vi "WCA_GET_PA.vi"(0 "Cartridge Band":u32=10, 1 "Slave Node in":cluster{"Address":i16, "Serial Number":i8[]}={"Address"=19, "Serial Number"=[16, 71, 55, 76, 1, 8, 0, -15]} {"Serial Number" format="%.0x"; "Address" format="%.0x"}, 2 "ObjHandle in":u32, 11 "error in (no error)":errorcluster) -> (4 "ObjHandle out":u32=92930112, 8 "GET_PA":T1={"PA_A_DRAIN_V"=0.0051879883, "PA_A_DRAIN_C"=3.829956, "PA_A_GATE_V"=-0.00061035156, "PA_B_DRAIN_V"=0.003967285, "PA_B_DRAIN_C"=4.4555664, "PA_B_GATE_V"=0.0018310547, "PA_3V_SUPPLY_V"=3.7371826, "PA_5V_MON"=5.310364}, 15 "error out":errorcluster)   [LabVIEW 2017]
uses:
  WCA_Global.vi
panel:
  # "Vd [V]"
  # "Id [mA]"
  # "Vg [V]"
  # "PA -3V Supply"
  # "-3V"
  # "PA A"
  # "+5V"
  # "PA B"
  # "Node Address"
  # "Serial Number"
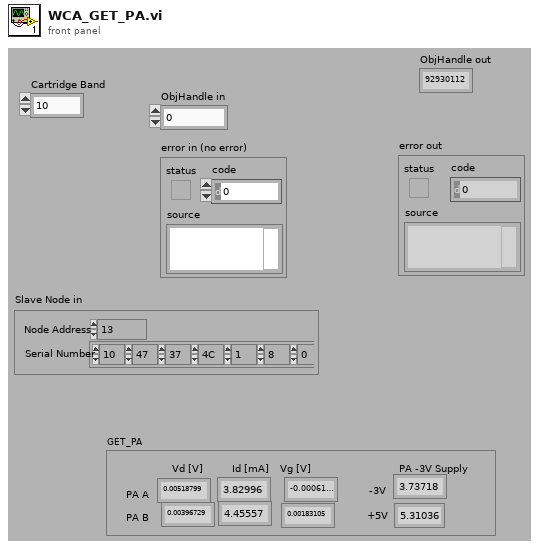
[diagram p1: front panel]
types:
  T1 = cluster{"PA_A_DRAIN_V":sgl, "PA_A_DRAIN_C":sgl, "PA_A_GATE_V":sgl, "PA_B_DRAIN_V":sgl, "PA_B_DRAIN_C":sgl, "PA_B_GATE_V":sgl, "PA_3V_SUPPLY_V":sgl, "PA_5V_MON":sgl}
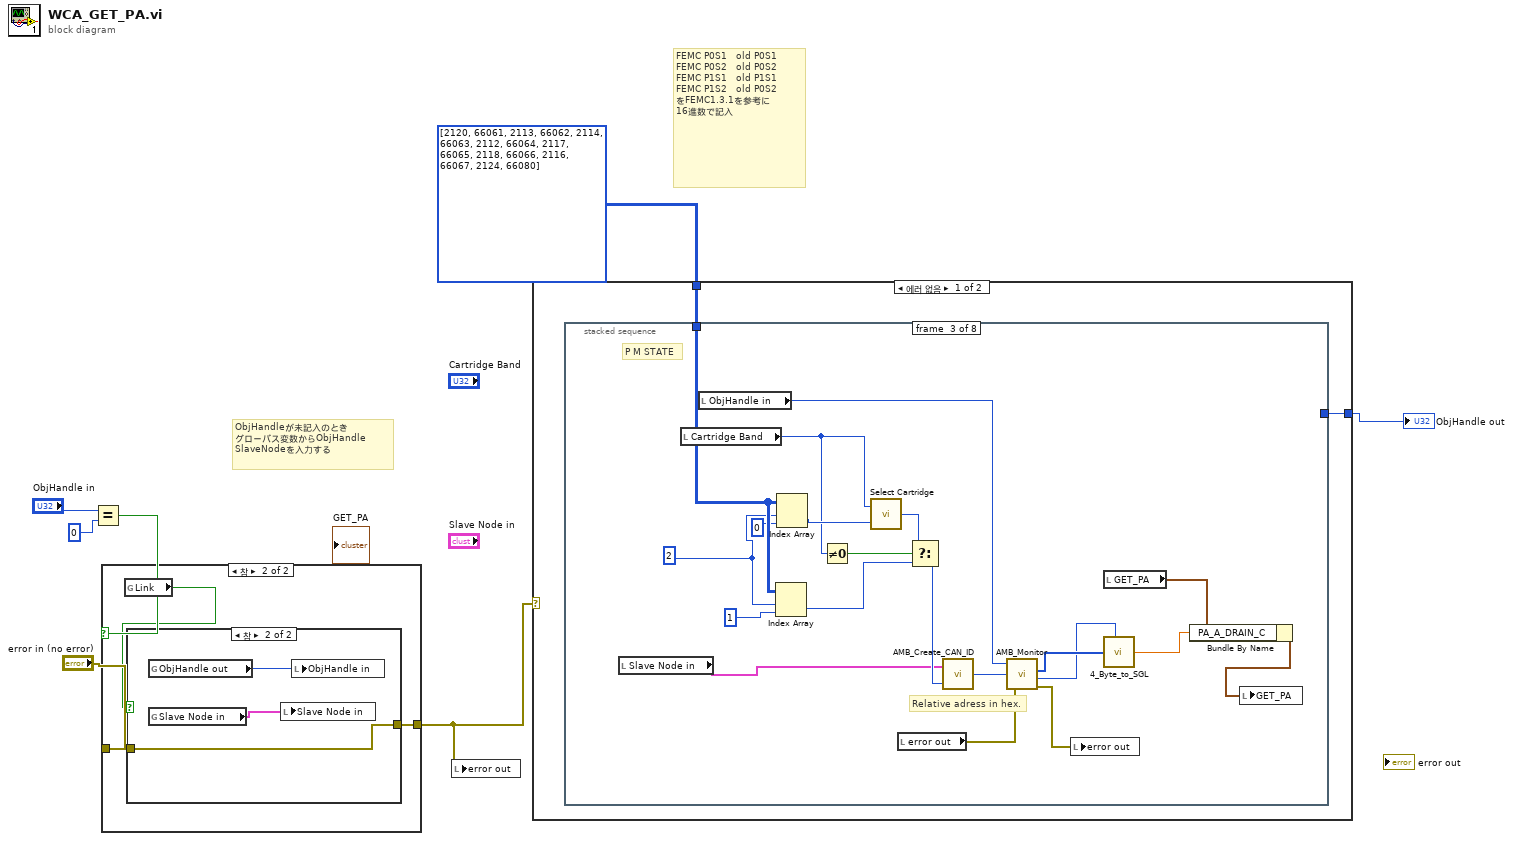
[diagram p0: block diagram]
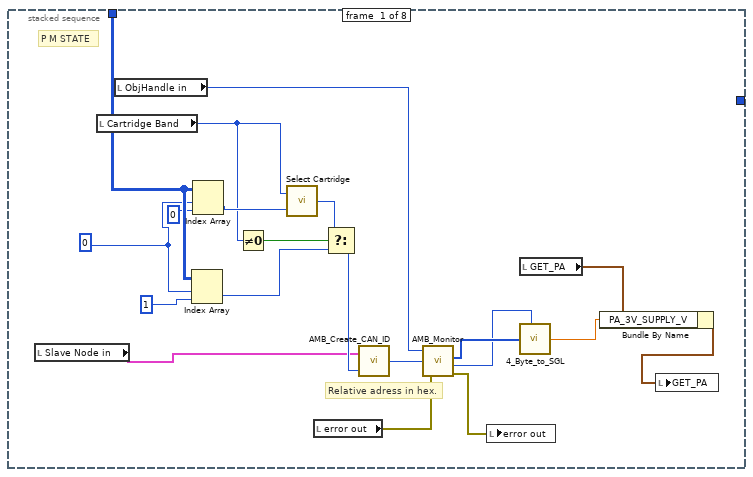
[diagram p2: hidden frame]
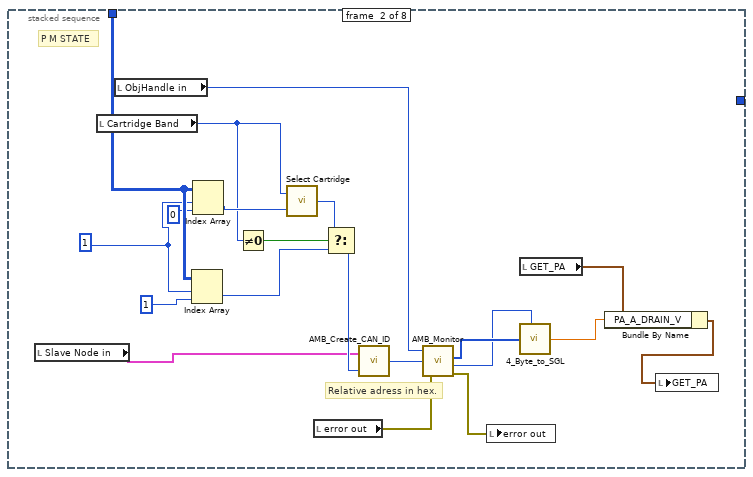
[diagram p3: hidden frame]
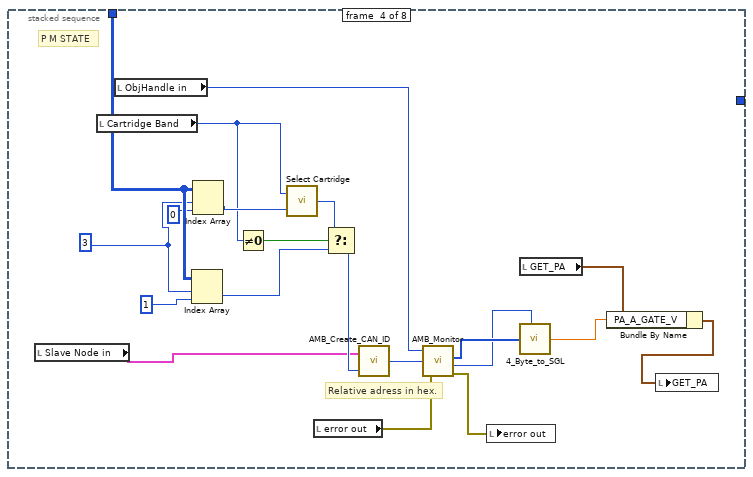
[diagram p4: hidden frame]
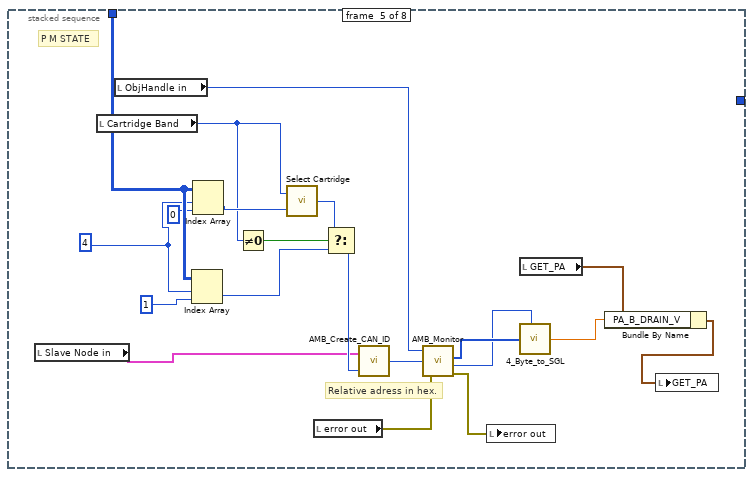
[diagram p5: hidden frame]
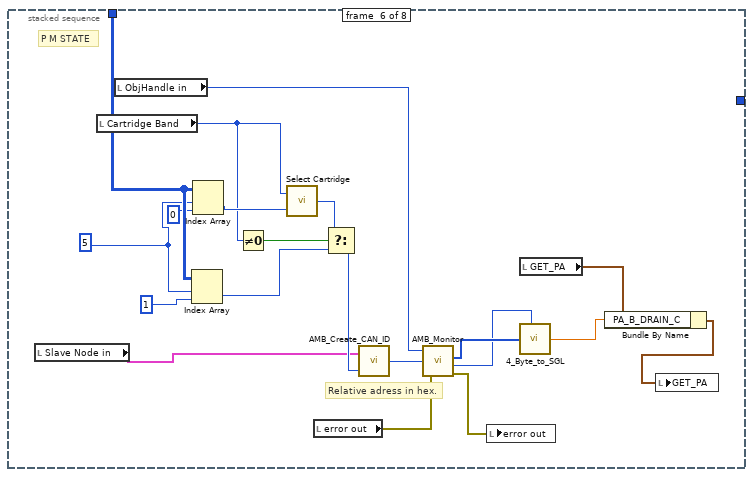
[diagram p6: hidden frame]
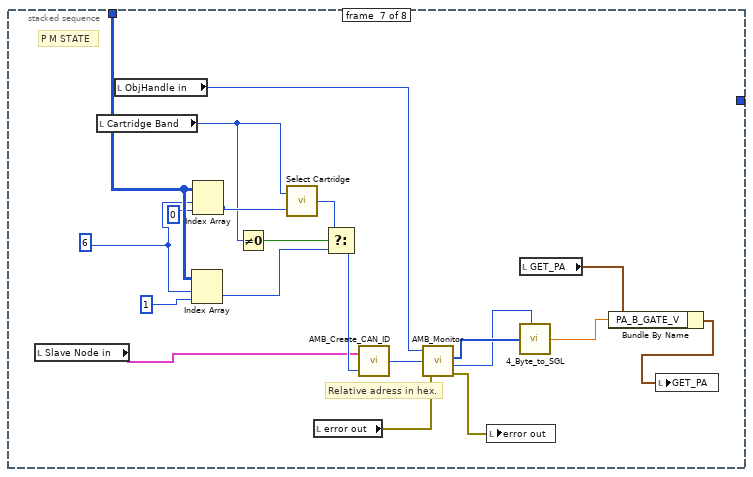
[diagram p7: hidden frame]
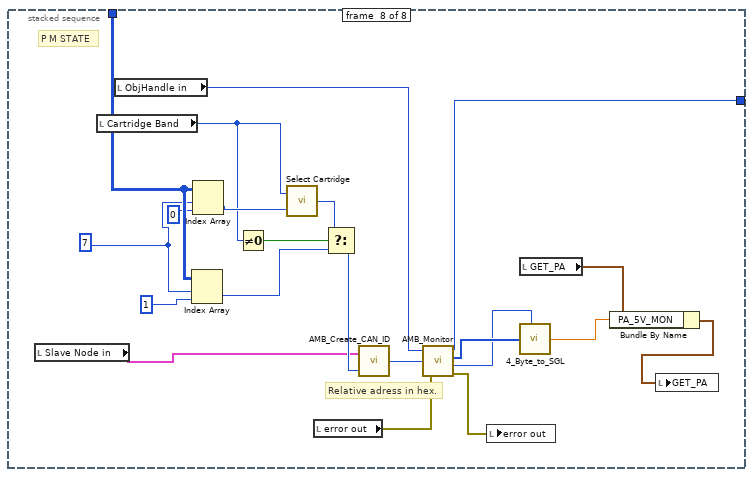
[diagram p8: hidden frame]
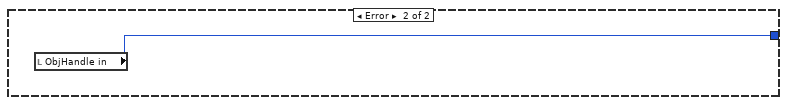
[diagram p9: hidden frame]
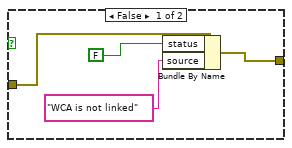
[diagram p11: hidden frame]
diagram:
  # "ObjHandleが未記入のとき\nグローバス変数からObjHandle\nSlaveNodeを入力する"
  # "FEMC P0S1   old P0S1\nFEMC P0S2   old P0S2\nFEMC P1S1   old P1S1\nFEMC P1S2   old P0S2\nをFEMC1.3.1を参考に\n16進数で記入"
  n1 = Equal?(x="ObjHandle in", y=0) -> (x = y?=w5:bool)
  n2 = case shown="참" w5 {
    tunnel: "error in (no error)" -> [w8 w11]
    tunnel: [w8 w10] -> w3
    frame False {
    }
    frame True {
      n3 = global read "WCA_Global.vi" "Link"() -> (w9:bool)
      n4 = case shown="참" w9 {
        tunnel: w11 -> [w15 w16]
        tunnel: [w12 w16] -> w10
        frame False {
          n5 = Bundle By Name(cluster=w15, "status"=FALSE, "source"="WCA is not linked") -> (w12:errorcluster)
        }
        frame True {
          n6 = global read "WCA_Global.vi" "ObjHandle out"() -> (w18:u32)
          n7 = global read "WCA_Global.vi" "Slave Node in"() -> (w17:cluster{"Address":i16, "Serial Number":i8[]})
          n8 = local write "Slave Node in"(w17) -> ()
          n9 = local write "ObjHandle in"(w18) -> ()
        }
      }
    }
  }
  n10 = local write "error out"(w3) -> ()
  n11 = case shown="에러 없음" w3 {
    tunnel: [w19 w182] -> w2
    tunnel: i32[][] [[2120, 66061], [2113, 66062], [2114, 66063], [2112, 66064], [2117, 66065], [2118, 66066], [2116, 66067], [2124, 66080]] -> [w20 _]
    frame No Error {
      n12 = stacked-sequence {
        tunnel: w20 -> [w40 w60 w80 w100 w120 w140 w160 w181]
        tunnel: [_ _ _ _ _ _ _ w161] -> w19
        frame #0 {
          w25 = 0
          # "Relative adress in hex."
          # "P M STATE"
          n13 = local read "Slave Node in"() -> (w24:cluster{"Address":i16, "Serial Number":i8[]})
          n14 = local read "Cartridge Band"() -> (w26:u32)
          n15 = local read "ObjHandle in"() -> (w36:u32)
          n16 = Index Array(array=w40, index (row)=w25, index (col)=1) -> (element=w35:i32)
          n17 = Index Array(array=w40, index (row)=w25, index (col)=0) -> (element=w34:i32)
          n18 = Not Equal To 0?(x=w26) -> (x != 0?=w37:bool)
          n19 = call "Select Cartridge.vi"("Relative Address in"=w34, "Cartridge band"=w26) -> ("Relative Address out"=w38:u32)
          n20 = local read "error out"() -> (w28:errorcluster)
          n21 = Select(t=w38, s=w37, f=w35) -> (s? t:f=w39:u32)
          n22 = call "AMB_Create_CAN_ID.vi"("Relative Address in"=w39, "Slave Node in"=w24) -> ("CAN ID out"=w31:u32)
          n23 = call "AMB_Monitor.vi"("ObjHandle in"=w36, "CAN ID in"=w31, "error in"=w28) -> ("Data Array out"=w23:u8[], "Data Length out"=w22:u8, "error out"=w27:errorcluster)  [unwired: 1 out]
          n24 = local write "error out"(w27) -> ()
          n25 = local read "GET_PA"() -> (w30:T1)
          n26 = call "4_Byte_to_SGL.vi"("Array of 4 bytes"=w23, "number of valid bytes"=w22) -> ("Number"=w21:sgl)  [unwired: 1 out]
          n27 = Bundle By Name(cluster=w30, "PA_3V_SUPPLY_V"=w21) -> (w29:T1)
          n28 = local write "GET_PA"(w29) -> ()
        }
        frame #1 {
          w45 = 1
          # "Relative adress in hex."
          # "P M STATE"
          n29 = local read "Slave Node in"() -> (w44:cluster{"Address":i16, "Serial Number":i8[]})
          n30 = local read "Cartridge Band"() -> (w46:u32)
          n31 = local read "ObjHandle in"() -> (w56:u32)
          n32 = Index Array(array=w60, index (row)=w45, index (col)=1) -> (element=w55:i32)
          n33 = Index Array(array=w60, index (row)=w45, index (col)=0) -> (element=w54:i32)
          n34 = Not Equal To 0?(x=w46) -> (x != 0?=w57:bool)
          n35 = call "Select Cartridge.vi"("Relative Address in"=w54, "Cartridge band"=w46) -> ("Relative Address out"=w58:u32)
          n36 = local read "error out"() -> (w48:errorcluster)
          n37 = Select(t=w58, s=w57, f=w55) -> (s? t:f=w59:u32)
          n38 = call "AMB_Create_CAN_ID.vi"("Relative Address in"=w59, "Slave Node in"=w44) -> ("CAN ID out"=w51:u32)
          n39 = call "AMB_Monitor.vi"("ObjHandle in"=w56, "CAN ID in"=w51, "error in"=w48) -> ("Data Array out"=w43:u8[], "Data Length out"=w42:u8, "error out"=w47:errorcluster)  [unwired: 1 out]
          n40 = local write "error out"(w47) -> ()
          n41 = local read "GET_PA"() -> (w50:T1)
          n42 = call "4_Byte_to_SGL.vi"("Array of 4 bytes"=w43, "number of valid bytes"=w42) -> ("Number"=w41:sgl)  [unwired: 1 out]
          n43 = Bundle By Name(cluster=w50, "PA_A_DRAIN_V"=w41) -> (w49:T1)
          n44 = local write "GET_PA"(w49) -> ()
        }
        frame #2 {
          w65 = 2
          # "Relative adress in hex."
          # "P M STATE"
          n45 = local read "Slave Node in"() -> (w64:cluster{"Address":i16, "Serial Number":i8[]})
          n46 = local read "Cartridge Band"() -> (w66:u32)
          n47 = local read "ObjHandle in"() -> (w76:u32)
          n48 = Index Array(array=w80, index (row)=w65, index (col)=1) -> (element=w75:i32)
          n49 = Index Array(array=w80, index (row)=w65, index (col)=0) -> (element=w74:i32)
          n50 = Not Equal To 0?(x=w66) -> (x != 0?=w77:bool)
          n51 = call "Select Cartridge.vi"("Relative Address in"=w74, "Cartridge band"=w66) -> ("Relative Address out"=w78:u32)
          n52 = local read "error out"() -> (w68:errorcluster)
          n53 = Select(t=w78, s=w77, f=w75) -> (s? t:f=w79:u32)
          n54 = call "AMB_Create_CAN_ID.vi"("Relative Address in"=w79, "Slave Node in"=w64) -> ("CAN ID out"=w71:u32)
          n55 = call "AMB_Monitor.vi"("ObjHandle in"=w76, "CAN ID in"=w71, "error in"=w68) -> ("Data Array out"=w63:u8[], "Data Length out"=w62:u8, "error out"=w67:errorcluster)  [unwired: 1 out]
          n56 = local write "error out"(w67) -> ()
          n57 = local read "GET_PA"() -> (w70:T1)
          n58 = call "4_Byte_to_SGL.vi"("Array of 4 bytes"=w63, "number of valid bytes"=w62) -> ("Number"=w61:sgl)  [unwired: 1 out]
          n59 = Bundle By Name(cluster=w70, "PA_A_DRAIN_C"=w61) -> (w69:T1)
          n60 = local write "GET_PA"(w69) -> ()
        }
        frame #3 {
          w85 = 3
          # "Relative adress in hex."
          # "P M STATE"
          n61 = local read "Slave Node in"() -> (w84:cluster{"Address":i16, "Serial Number":i8[]})
          n62 = local read "Cartridge Band"() -> (w86:u32)
          n63 = local read "ObjHandle in"() -> (w96:u32)
          n64 = Index Array(array=w100, index (row)=w85, index (col)=1) -> (element=w95:i32)
          n65 = Index Array(array=w100, index (row)=w85, index (col)=0) -> (element=w94:i32)
          n66 = Not Equal To 0?(x=w86) -> (x != 0?=w97:bool)
          n67 = call "Select Cartridge.vi"("Relative Address in"=w94, "Cartridge band"=w86) -> ("Relative Address out"=w98:u32)
          n68 = local read "error out"() -> (w88:errorcluster)
          n69 = Select(t=w98, s=w97, f=w95) -> (s? t:f=w99:u32)
          n70 = call "AMB_Create_CAN_ID.vi"("Relative Address in"=w99, "Slave Node in"=w84) -> ("CAN ID out"=w91:u32)
          n71 = call "AMB_Monitor.vi"("ObjHandle in"=w96, "CAN ID in"=w91, "error in"=w88) -> ("Data Array out"=w83:u8[], "Data Length out"=w82:u8, "error out"=w87:errorcluster)  [unwired: 1 out]
          n72 = local write "error out"(w87) -> ()
          n73 = local read "GET_PA"() -> (w90:T1)
          n74 = call "4_Byte_to_SGL.vi"("Array of 4 bytes"=w83, "number of valid bytes"=w82) -> ("Number"=w81:sgl)  [unwired: 1 out]
          n75 = Bundle By Name(cluster=w90, "PA_A_GATE_V"=w81) -> (w89:T1)
          n76 = local write "GET_PA"(w89) -> ()
        }
        frame #4 {
          w105 = 4
          # "Relative adress in hex."
          # "P M STATE"
          n77 = local read "Slave Node in"() -> (w104:cluster{"Address":i16, "Serial Number":i8[]})
          n78 = local read "Cartridge Band"() -> (w106:u32)
          n79 = local read "ObjHandle in"() -> (w116:u32)
          n80 = Index Array(array=w120, index (row)=w105, index (col)=1) -> (element=w115:i32)
          n81 = Index Array(array=w120, index (row)=w105, index (col)=0) -> (element=w114:i32)
          n82 = Not Equal To 0?(x=w106) -> (x != 0?=w117:bool)
          n83 = call "Select Cartridge.vi"("Relative Address in"=w114, "Cartridge band"=w106) -> ("Relative Address out"=w118:u32)
          n84 = local read "error out"() -> (w108:errorcluster)
          n85 = Select(t=w118, s=w117, f=w115) -> (s? t:f=w119:u32)
          n86 = call "AMB_Create_CAN_ID.vi"("Relative Address in"=w119, "Slave Node in"=w104) -> ("CAN ID out"=w111:u32)
          n87 = call "AMB_Monitor.vi"("ObjHandle in"=w116, "CAN ID in"=w111, "error in"=w108) -> ("Data Array out"=w103:u8[], "Data Length out"=w102:u8, "error out"=w107:errorcluster)  [unwired: 1 out]
          n88 = local write "error out"(w107) -> ()
          n89 = local read "GET_PA"() -> (w110:T1)
          n90 = call "4_Byte_to_SGL.vi"("Array of 4 bytes"=w103, "number of valid bytes"=w102) -> ("Number"=w101:sgl)  [unwired: 1 out]
          n91 = Bundle By Name(cluster=w110, "PA_B_DRAIN_V"=w101) -> (w109:T1)
          n92 = local write "GET_PA"(w109) -> ()
        }
        frame #5 {
          w125 = 5
          # "Relative adress in hex."
          # "P M STATE"
          n93 = local read "Slave Node in"() -> (w124:cluster{"Address":i16, "Serial Number":i8[]})
          n94 = local read "Cartridge Band"() -> (w126:u32)
          n95 = local read "ObjHandle in"() -> (w136:u32)
          n96 = Index Array(array=w140, index (row)=w125, index (col)=1) -> (element=w135:i32)
          n97 = Index Array(array=w140, index (row)=w125, index (col)=0) -> (element=w134:i32)
          n98 = Not Equal To 0?(x=w126) -> (x != 0?=w137:bool)
          n99 = call "Select Cartridge.vi"("Relative Address in"=w134, "Cartridge band"=w126) -> ("Relative Address out"=w138:u32)
          n100 = local read "error out"() -> (w128:errorcluster)
          n101 = Select(t=w138, s=w137, f=w135) -> (s? t:f=w139:u32)
          n102 = call "AMB_Create_CAN_ID.vi"("Relative Address in"=w139, "Slave Node in"=w124) -> ("CAN ID out"=w131:u32)
          n103 = call "AMB_Monitor.vi"("ObjHandle in"=w136, "CAN ID in"=w131, "error in"=w128) -> ("Data Array out"=w123:u8[], "Data Length out"=w122:u8, "error out"=w127:errorcluster)  [unwired: 1 out]
          n104 = local write "error out"(w127) -> ()
          n105 = local read "GET_PA"() -> (w130:T1)
          n106 = call "4_Byte_to_SGL.vi"("Array of 4 bytes"=w123, "number of valid bytes"=w122) -> ("Number"=w121:sgl)  [unwired: 1 out]
          n107 = Bundle By Name(cluster=w130, "PA_B_DRAIN_C"=w121) -> (w129:T1)
          n108 = local write "GET_PA"(w129) -> ()
        }
        frame #6 {
          w145 = 6
          # "Relative adress in hex."
          # "P M STATE"
          n109 = local read "Slave Node in"() -> (w144:cluster{"Address":i16, "Serial Number":i8[]})
          n110 = local read "Cartridge Band"() -> (w146:u32)
          n111 = local read "ObjHandle in"() -> (w156:u32)
          n112 = Index Array(array=w160, index (row)=w145, index (col)=1) -> (element=w155:i32)
          n113 = Index Array(array=w160, index (row)=w145, index (col)=0) -> (element=w154:i32)
          n114 = Not Equal To 0?(x=w146) -> (x != 0?=w157:bool)
          n115 = call "Select Cartridge.vi"("Relative Address in"=w154, "Cartridge band"=w146) -> ("Relative Address out"=w158:u32)
          n116 = local read "error out"() -> (w148:errorcluster)
          n117 = Select(t=w158, s=w157, f=w155) -> (s? t:f=w159:u32)
          n118 = call "AMB_Create_CAN_ID.vi"("Relative Address in"=w159, "Slave Node in"=w144) -> ("CAN ID out"=w151:u32)
          n119 = call "AMB_Monitor.vi"("ObjHandle in"=w156, "CAN ID in"=w151, "error in"=w148) -> ("Data Array out"=w143:u8[], "Data Length out"=w142:u8, "error out"=w147:errorcluster)  [unwired: 1 out]
          n120 = local write "error out"(w147) -> ()
          n121 = local read "GET_PA"() -> (w150:T1)
          n122 = call "4_Byte_to_SGL.vi"("Array of 4 bytes"=w143, "number of valid bytes"=w142) -> ("Number"=w141:sgl)  [unwired: 1 out]
          n123 = Bundle By Name(cluster=w150, "PA_B_GATE_V"=w141) -> (w149:T1)
          n124 = local write "GET_PA"(w149) -> ()
        }
        frame #7 {
          w166 = 7
          # "Relative adress in hex."
          # "P M STATE"
          n125 = local read "Slave Node in"() -> (w165:cluster{"Address":i16, "Serial Number":i8[]})
          n126 = local read "Cartridge Band"() -> (w167:u32)
          n127 = local read "ObjHandle in"() -> (w177:u32)
          n128 = Index Array(array=w181, index (row)=w166, index (col)=1) -> (element=w176:i32)
          n129 = Index Array(array=w181, index (row)=w166, index (col)=0) -> (element=w175:i32)
          n130 = Not Equal To 0?(x=w167) -> (x != 0?=w178:bool)
          n131 = call "Select Cartridge.vi"("Relative Address in"=w175, "Cartridge band"=w167) -> ("Relative Address out"=w179:u32)
          n132 = local read "error out"() -> (w169:errorcluster)
          n133 = Select(t=w179, s=w178, f=w176) -> (s? t:f=w180:u32)
          n134 = call "AMB_Create_CAN_ID.vi"("Relative Address in"=w180, "Slave Node in"=w165) -> ("CAN ID out"=w172:u32)
          n135 = call "AMB_Monitor.vi"("ObjHandle in"=w177, "CAN ID in"=w172, "error in"=w169) -> ("ObjHandle out"=w161:u32, "Data Array out"=w164:u8[], "Data Length out"=w163:u8, "error out"=w168:errorcluster)
          n136 = local write "error out"(w168) -> ()
          n137 = local read "GET_PA"() -> (w171:T1)
          n138 = call "4_Byte_to_SGL.vi"("Array of 4 bytes"=w164, "number of valid bytes"=w163) -> ("Number"=w162:sgl)  [unwired: 1 out]
          n139 = Bundle By Name(cluster=w171, "PA_5V_MON"=w162) -> (w170:T1)
          n140 = local write "GET_PA"(w170) -> ()
        }
      }
    }
    frame Error {
      n141 = local read "ObjHandle in"() -> (w182:u32)
    }
  }
  "ObjHandle out" <- w2
